vi "test - datatype cacher.vi"() -> ()   [LabVIEW 2017]
uses:
  <vilib>/Utility/Data Type/Type Definitions/Data Type.ctl
  String/_Support/DataType Cacher(Data).vi
  <vilib>/Utility/Data Type/Get Type Information.vi
  String/_Support/DataType Cacher(DT).vi
  <vilib>/Utility/Data Type/NI_Data Type.lvlib
panel:
  out "should not error":errorcluster
  out "cacher 3":variant
  out "match? 3":bool
  out "stored type 3":T1
  out "Data(Dup) 3":variant
  out "cacher 2":variant
  out "match? 2":bool
  out "stored type 2":T1
  out "Data(Dup) 2":variant
  out "cacher":variant
  out "match?":bool
  out "stored type":T1
  out "Data(Dup)":variant
  out "EXPECETED ERROR":errorcluster
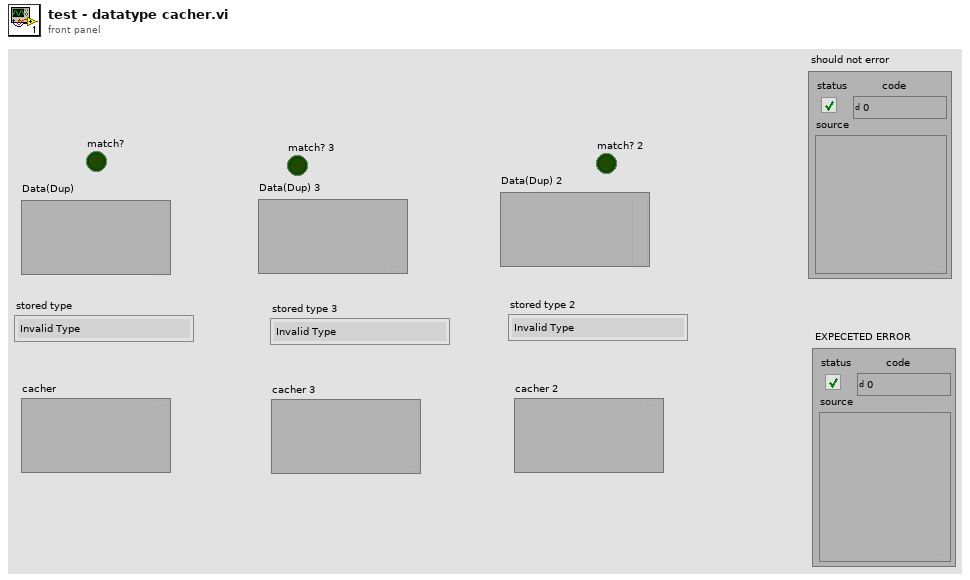
[diagram p1: front panel]
types:
  T1 = typedef "NI_Data Type.lvlib/Data Type.ctl" = enum8{"Invalid Type", "Void", "I8", "I16", "I32", "I64", "U8", "U16", "U32", "U64", "Single Float", "Double Float", "Extended Float", "Single Complex", "Double Complex", "Extended Complex", "Enum U8", "Enum U16", "Enum U32", "Enum U64", "Single Float With Unit", "Double Float With Unit", "Extended Float With Unit", "Single Complex with Unit", "Double Complex with Unit", "Extended Complex with Unit", "Boolean", "String", "Path", "Picture", "Tag", "Array", "Cluster", "Variant", "LV Variant", "Waveform", "Timestamp", "Digital Waveform", "Digital Data", "ExpressData", "Refnum", "External Data", "VI", "Poly VI", "LabVIEW Class Instance", "Fixed Point"}
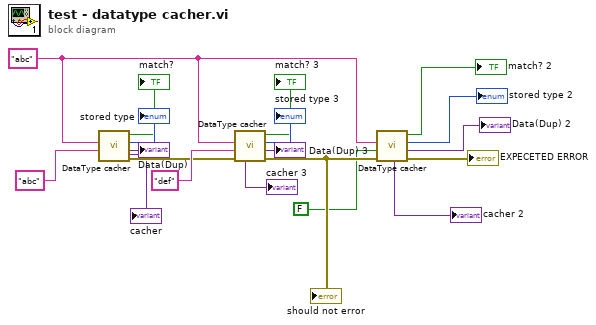
[diagram p0: block diagram]
diagram:
  w14 = "abc"
  n1 = call-poly "DataType cacher.vi"("Data"="abc", "key(use dataname if empty)"=w14) -> ("error out"=w13:errorcluster, "Data(Dup)"=→"Data(Dup)":variant, "stored type"=→"stored type":T1, "match?"=→"match?":bool, "cacher"=→"cacher":variant)  [unwired: 5 in]
  n2 = call-poly "DataType cacher.vi"("error in (no error)"=w13, "Data"="def", "key(use dataname if empty)"=w14) -> ("error out"=w18:errorcluster, "Data(Dup)"=→"Data(Dup) 3":variant, "stored type"=→"stored type 3":T1, "match?"=→"match? 3":bool, "cacher"=→"cacher 3":variant)  [unwired: 4 in]
  "should not error" <- w18
  n3 = call-poly "DataType cacher.vi"("error in (no error)"=w18, "Data"=FALSE, "key(use dataname if empty)"=w14) -> ("error out"=→"EXPECETED ERROR":errorcluster, "Data(Dup)"=→"Data(Dup) 2":variant, "stored type"=→"stored type 2":T1, "match?"=→"match? 2":bool, "cacher"=→"cacher 2":variant)  [unwired: 4 in]
